vi "LatLongEmpty.vi"(8 "error (in)":errorcluster, 10 "GPS Data":T7, 11 "LINX Resource":T1) -> (0 "error (out)":errorcluster, 1 "Empty or not in range?":bool, 2 "GPS Data":T7, 3 "LINX Resource":T1)   [LabVIEW 2015]
doc: "Has the GPS fixed a current location?"
uses:
  <vilib>/MakerHub/LINX/Private/Type Defs/LINX Ref.ctl
  <vilib>/MakerHub/LINX/Private/Type Defs/Platform.ctl
  <vilib>/MakerHub/LINX/Private/Type Defs/Interface.ctl
  <vilib>/MakerHub/LINX/Private/Device/Type Defs/LINX Device Config.ctl
  <vilib>/MakerHub/LINX/Private/Device/Type Defs/TCP Config.ctl
  <vilib>/MakerHub/LINX/Private/Device/Type Defs/Channels.ctl
  <vilib>/MakerHub/LINX/LMH-LINX.lvlib
  <vilib>/MakerHub/LINX/Private/Device/Device.lvlib
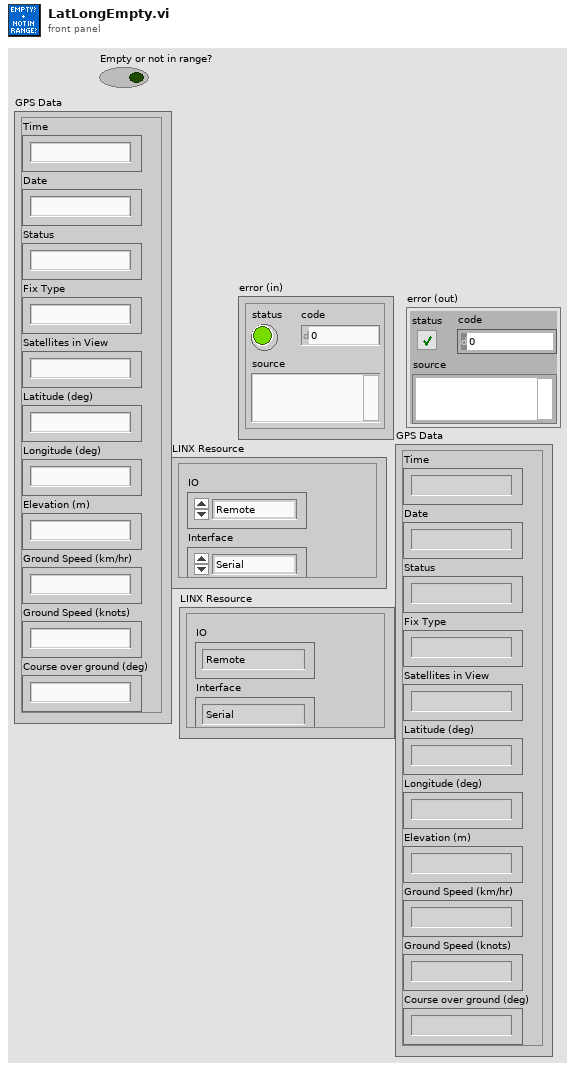
[diagram p1: front panel]
types:
  T1 = typedef "LMH-LINX.lvlib/LINX Ref.ctl" = cluster{"IO":T2, "Interface":T3, "LINX Device Config":T4}
  T2 = typedef "LMH-LINX.lvlib/Platform.ctl" = enum16{"Remote", "Local"}
  T3 = typedef "LMH-LINX.lvlib/Interface.ctl" = enum16{"Serial", "TCP"}
  T4 = typedef "LMH-LINX.lvlib/Device.lvlib/LINX Device Config.ctl" = cluster{"Interface":T3, "COM Port":refnum<visa-resource-name>, "TCP Configuration":T5, "Device Family":u8, "Device ID":u8, "Device Name":string, "TCP Ref":refnum<k5>, "Channels":T6}
  T5 = typedef "LMH-LINX.lvlib/Device.lvlib/TCP Config.ctl" = cluster{"IP Address":string, "Port":u16}
  T6 = typedef "LMH-LINX.lvlib/Channels.ctl" = cluster{"DI":u8[], "DO":u8[], "AI":u8[], "AO":u8[], "PWM":u8[], "QE":u8[], "UART":u8[], "I2C 2":u8[], "SPI":u8[], "CAN":u8[], "Servo":u8[], "AI Ref (V)":dbl, "AI Resolution (Bits)":u8, "AO Ref (V)":dbl, "AO Resolution (Bits)":u8}
  T7 = cluster{"Time":string, "Date":string, "Status":string, "Fix Type":string, "Satellites in View":string, "Latitude (deg)":string, "Longitude (deg)":string, "Elevation (m)":string, "Ground Speed (km/hr)":string, "Ground Speed (knots)":string, "Course over ground (deg)":string}
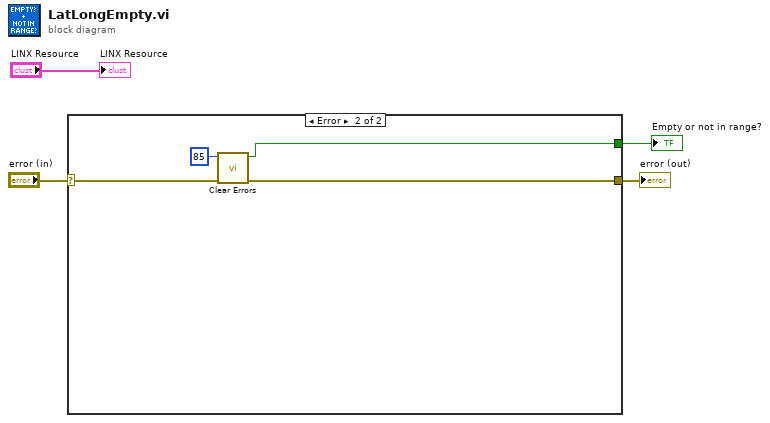
[diagram p0: block diagram]
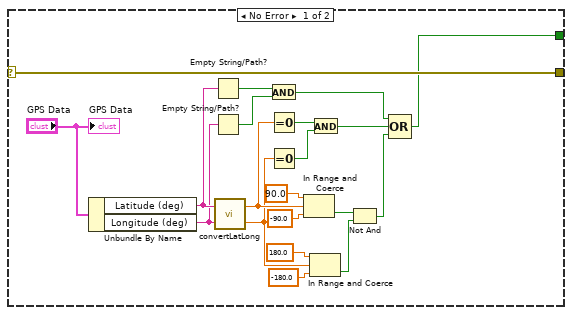
[diagram p2: hidden frame]
diagram:
  n1 = case shown="Error" "error (in)" {
    selector: "error (in)" -> [w15 w28]
    tunnel: [w15 w27] -> w3
    tunnel: [w5 w26] -> w1
    frame No Error {
      n2 = Unbundle By Name("GPS Data") -> ("Latitude (deg)"=w21:string, "Longitude (deg)"=w20:string)
      n3 = Empty String/Path?(string/path=w21) -> (empty?=w24:bool)
      n4 = Empty String/Path?(string/path=w20) -> (empty?=w23:bool)
      n5 = call "convertLatLong.vi"("Longitude (deg)"=w20, "Latitude (deg)"=w21) -> ("Longitude (deg)"=w11:dbl, "Latitude (deg)"=w14:dbl)
      n6 = And(x=w24, y=w23) -> (x .and. y?=w17:bool)
      n7 = Equal To 0?(x=w14) -> (x = 0?=w19:bool)
      n8 = Equal To 0?(x=w11) -> (x = 0?=w18:bool)
      n9 = In Range and Coerce(upper limit=90.0, x=w14, lower limit=-90.0) -> (In Range?=w8:bool)  [unwired: 1 out]
      n10 = In Range and Coerce(upper limit=180.0, x=w11, lower limit=-180.0) -> (In Range?=w7:bool)  [unwired: 1 out]
      n11 = And(x=w19, y=w18) -> (x .and. y?=w16:bool)
      n12 = Not And(1:w7, 2:w8) -> (0:w6:bool)
      n13 = Compound Arithmetic op=OR(w17, w16, w6) -> (w5:bool)
      "GPS Data" <- "GPS Data"
    }
    frame Error {
      n14 = call <vilib>:"Clear Errors.vi"("error in (no error)"=w28, "specific error code to clear (0: all)"=85) -> ("error out"=w27:errorcluster, "specific error cleared?"=w26:bool)  [unwired: 4 in]
    }
  }
  "error (out)" <- w3
  "Empty or not in range?" <- w1
  "LINX Resource" <- "LINX Resource"
